vi "Configure Channel Offset.vi.vi"(8 "error in (no error)":errorcluster, 9 "Channel Offset (0 dB)":dbl, 10 "Enable Channel Offset (F: Disable)":bool, 11 "VISA resource name":refnum<visa-resource-name>) -> (0 "error out":errorcluster, 3 "VISA resource name out":refnum<visa-resource-name>)   [LabVIEW 2011, in "Agilent N432A.lvlib"]
doc: "Configures the channel offset value. Channel offset is applied to the measured power before any mathematical functions display offsets, or relative functions are included."
uses:
  <instrlib>/Agilent N432A/Agilent N432A.lvlib
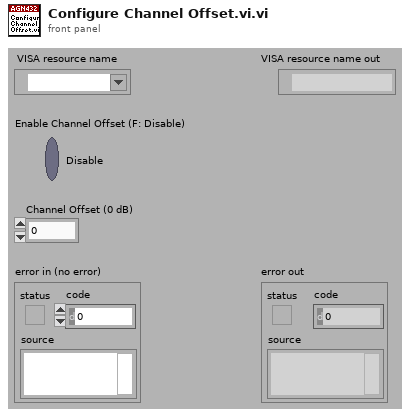
[diagram p1: front panel]
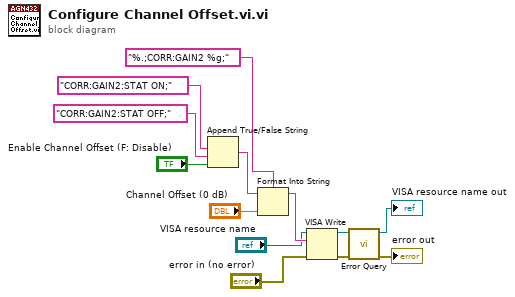
[diagram p0: block diagram]
diagram:
  n1 = Append True/False String(1:"Enable Channel Offset (F: Disable)", 2:"CORR:GAIN2:STAT OFF;", 3:"CORR:GAIN2:STAT ON;") -> (0:w10:string)  [unwired: 1 in]
  n2 = Format Into String(format string="%.;CORR:GAIN2 %g;", initial string=w10, "Channel Offset (0 dB)") -> (resulting string=w7:string)  [unwired: 1 in, 1 out]
  n3 = VISA Write(VISA resource name="VISA resource name", write buffer=w7, error in (no error)="error in (no error)") -> (VISA resource name out=w4:refnum<visa-resource-name>, error out=w3:errorcluster)  [unwired: 1 out]
  n4 = call <instrlib>:"Error Query.vi"("error in (no error)"=w3, "VISA resource name"=w4) -> ("error out"=→"error out":errorcluster, "VISA resource name out"=→"VISA resource name out":refnum<visa-resource-name>)  [unwired: 6 in, 2 out]
